vi "get data from HW.vi"() -> ()   [LabVIEW 2017]
uses:
  Control/Config chanel.ctl
  <vilib>/DAQmx/create/channels.llb/DAQmx Create Channel (AI-Voltage-Basic).vi
  <vilib>/DAQmx/configure/timing.llb/DAQmx Timing (Sample Clock).vi
  <vilib>/DAQmx/read.llb/DAQmx Read (Analog 1D Wfm NChan NSamp).vi
  <vilib>/measure/NI_MAPro.lvlib
  <vilib>/measure/matone.llb/Extract Single Tone Information 1 Chan.vi
panel:
  out "detected frequency":dbl format="%.2p"
  in  "stop":bool
  out "Waveform Chart":waveform(dbl)[](graph)
  in  "DAQ Config":T1
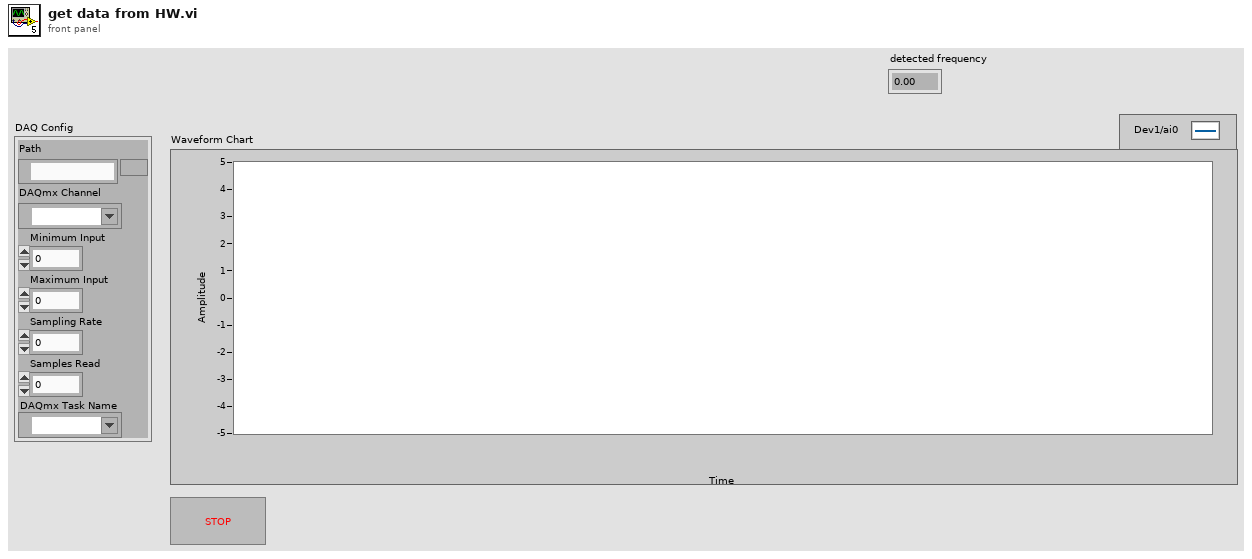
[diagram p1: front panel]
types:
  T1 = typedef "Config chanel.ctl" = cluster{"Path":path, "DAQmx Channel":tag, "Minimum Input":dbl, "Maximum Input":dbl, "Sampling Rate":dbl, "Samples Read":dbl, "DAQmx Task Name":refnum<k21>}
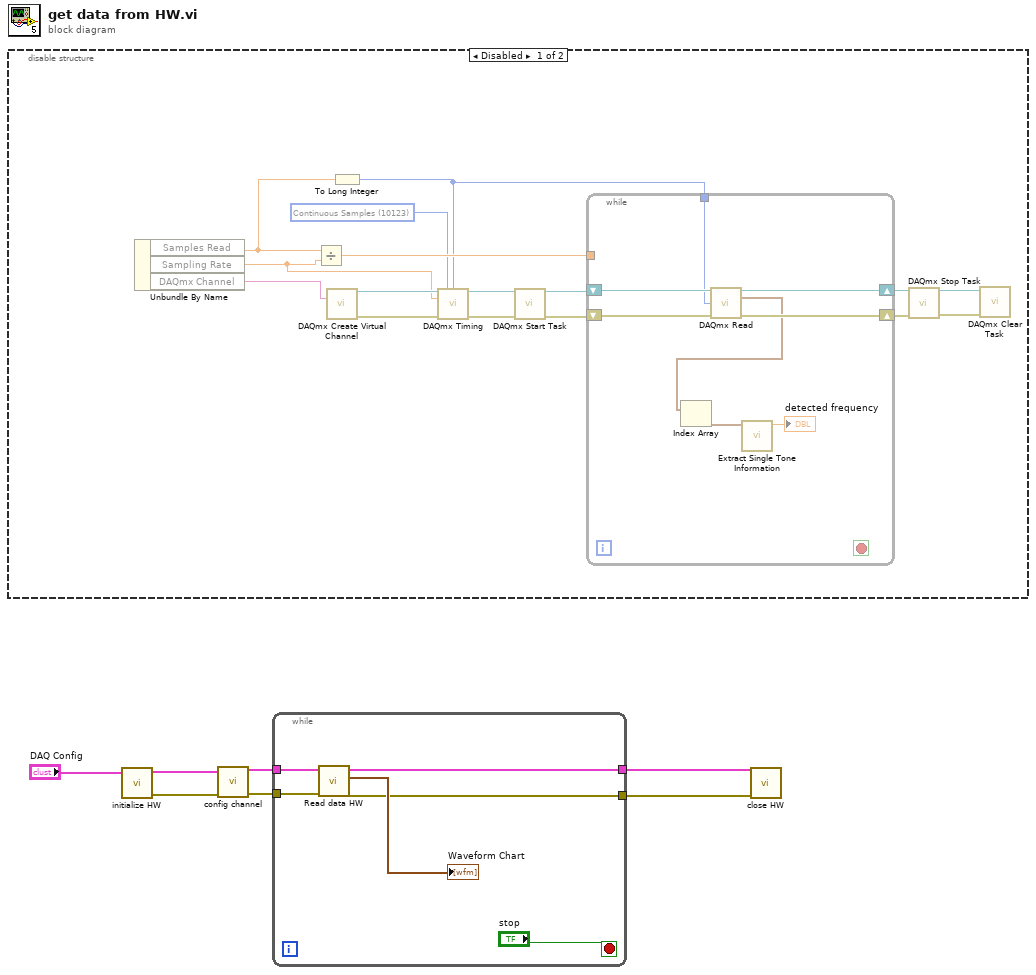
[diagram p0: block diagram]
diagram:
  n1 = disable-structure shown="Disabled" {
    frame Disabled {
      w15 = 10123 items=["Finite Samples"=10178, "Continuous Samples"=10123, "Hardware Timed Single Point"=12522] ("sample mode")
      n2 = Unbundle By Name() -> ("Samples Read"=w14:dbl, "Sampling Rate"=w16:dbl, "DAQmx Channel"=w8:tag)  [unwired: 1 in]
      n3 = Divide(x=w14, y=w16) -> (x/y=w17:dbl)
      n4 = call-poly <vilib>:"DAQmx Create Virtual Channel.vi"("physical channels"=w8) -> ("task out"=w23:refnum<k21>, "error out"=w22:errorcluster)  [unwired: 13 in]
      n5 = To Long Integer(number=w14) -> (32bit integer=w9:i32)
      n6 = call-poly <vilib>:"DAQmx Timing.vi"("task/channels in"=w23, "sample mode"=w15, "samples per channel"=w9, "rate"=w16, "error in"=w22) -> ("task out"=w13:refnum<k21>, "error out"=w12:errorcluster)  [unwired: 9 in]
      n7 = call <vilib>:"DAQmx Start Task.vi"("task/channels in"=w13, "error in"=w12) -> ("task out"=w11:refnum<k21>, "error out"=w10:errorcluster)  [unwired: 12 in]
      n8 = while {
        shift-right: [w31] -> w21
        shift-left: w11 -> [w29]
        shift-right: [w30] -> w20
        shift-left: w10 -> [w28]
        tunnel: w17 -> [_]
        tunnel: w9 -> [w27]
        stop <- _ stop-if-true
        n9 = call-poly <vilib>:"DAQmx Read.vi"("task/channels in"=w29, "number of samples per channel"=w27, "error in"=w28) -> ("task out"=w31:refnum<k21>, "data"=w26:waveform(dbl)[], "error out"=w30:errorcluster)  [unwired: 10 in]
        n10 = Index Array(array=w26) -> (element=w25:waveform(dbl))  [unwired: 1 in]
        n11 = call-poly <vilib>:"Extract Single Tone Information.vi"("time signal in"=w25) -> ("detected frequency"=→"detected frequency":dbl)  [unwired: 5 in, 5 out]
      }
      n12 = call <vilib>:"DAQmx Stop Task.vi"("task/channels in"=w21, "error in"=w20) -> ("task out"=w18:refnum<k21>, "error out"=w19:errorcluster)  [unwired: 12 in]
      n13 = call <vilib>:"DAQmx Clear Task.vi"("task in"=w18, "error in"=w19) -> ()  [unwired: 13 in, 1 out]
    }
    frame Enabled {
    }
  }
  n14 = call "initialize HW.vi"("DAQ Config"="DAQ Config") -> ("error out"=w5:errorcluster, "DAQ Config out"=w6:T1)  [unwired: 9 in]
  n15 = call "config channel.vi"("error in"=w5, "DAQ Config"=w6) -> ("error out"=w3:errorcluster, "DAQ Config out"=w4:T1)  [unwired: 8 in]
  n16 = while {
    tunnel: w4 -> [w37]
    tunnel: w3 -> [w36]
    tunnel: [w34] -> w2
    tunnel: [w33] -> w1
    stop <- "stop" stop-if-true
    n17 = call "Read data HW.vi"("error in"=w36, "HW Resource in"=w37) -> ("error out"=w33:errorcluster, "data"=→"Waveform Chart":waveform(dbl)[], "HW Resource out"=w34:T1)  [unwired: 7 in]
  }
  n18 = call "close HW.vi"("error in"=w1, "DAQ Config"=w2) -> ()  [unwired: 9 in, 1 out]
